vi "Periodic Tasks.vi"(8 "error in":errorcluster) -> ()   [LabVIEW 2013]
doc: "This VI runs in parallel to other tasks. It can contain as many user-defined periodic loops as you need. These can carry out PID or other sorts of timed response."
uses:
  <vilib>/Rock Robotics/WPI/Relay/WPI_RelayValue.ctl
  <vilib>/vision/Image Controls.llb/IMAQ Image.ctl
  <vilib>/Rock Robotics/SystemInterfaces/Utilities/FPGA_UtilitiesLED Source.ctl
  <vilib>/Rock Robotics/SystemInterfaces/Utilities/FPGA_UtilitiesLED State.ctl
  <vilib>/Rock Robotics/WPI/Solenoid/WPI_SolenoidValue.ctl
  Robot Global Data.vi
  <vilib>/Rock Robotics/WPI/Solenoid/WPI_SolenoidSetEnum.vi
  <vilib>/Rock Robotics/WPI/Joystick/WPI_JoystickGetSetRefNum.vi
  <vilib>/Rock Robotics/WPI/Solenoid/WPI_SolenoidGetEnum.vi
  <vilib>/Rock Robotics/WPI/Compressor/WPI_CompressorGetSetRefNum.vi
panel:
  out "Distance":dbl
  out "Rate 2":dbl
  out "Rate":dbl
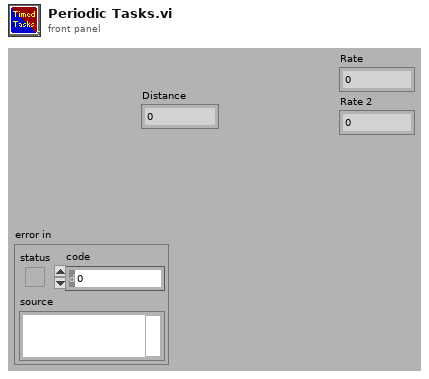
[diagram p1: front panel]
types:
  T1 = typedef "FPGA_UtilitiesLED State.ctl" = enum16{"Off", "On", "Toggle"}
  T2 = typedef "FPGA_UtilitiesLED Source.ctl" = enum16{"User LED", "FPGA LED"}
  T3 = typedef "WPI_DigitalInputDevRef.ctl" = cluster{"DevStatus":errorcluster, "DIO Channel":T4, "Digital Module":T5}
  T4 = typedef "FPGA_DIOChannel.ctl" = enum8{"DIO 1", "DIO 2", "DIO 3", "DIO 4", "DIO 5", "DIO 6", "DIO 7", "DIO 8", "DIO 9", "DIO 10", "DIO 11", "DIO 12", "DIO 13", "DIO 14", "Invalid"}
  T5 = typedef "FPGA_TypedefDigitalModule.ctl" = enum16{"Digital Module 1", "Digital Module 2"}
  T6 = typedef "WPI_SolenoidDevRef.ctl" = cluster{"DevStatus":errorcluster, "Solenoid Module":T7, "Forward Solenoid Channel":T8, "Reverse Solenoid Channel":T8}
  T7 = typedef "FPGA_TypedefSolenoidModule.ctl" = enum16{"Solenoid Module 1", "Solenoid Module 2"}
  T8 = typedef "WPI_SolenoidChannel.ctl" = enum8{"Solenoid 1", "Solenoid 2", "Solenoid 3", "Solenoid 4", "Solenoid 5", "Solenoid 6", "Solenoid 7", "Solenoid 8", "Invalid"}
  T9 = typedef "WPI_EncoderDevRef.ctl" = cluster{"DevStatus":errorcluster, "EncoderIndex":T10, "CounterIndex":T11, "DistancePerCount":dbl, "Decoding Type":T12}
  T10 = typedef "FPGA_EncoderIdx.ctl" = enum8{"Enc 0", "Enc 1", "Enc 2", "Enc 3", "Invalid"}
  T11 = typedef "FPGA_CounterCtrSystemIndex.ctl" = enum8{"Ctr 0", "Ctr 1", "Ctr 2", "Ctr 3", "Ctr 4", "Ctr 5", "Ctr 6", "Ctr 7", "Invalid"}
  T12 = typedef "WPI_EncoderType.ctl" = enum16{"1x", "2x", "4x"}
  T13 = typedef "WPI_JoystickDevRef.ctl" = cluster{"Device":T14}
  T14 = typedef "WPI_JoystickDeviceEnum.ctl" = enum16{"USB 1", "USB 2", "USB 3", "USB 4", "Kinect 1", "Kinect 2"}
  T15 = typedef "WPI_CompressorDevRef.ctl" = cluster{"DevStatus":errorcluster, "DigitalInputDevRef":T3, "RelayDevRef":T16}
  T16 = typedef "WPI_RelayDevRef.ctl" = cluster{"DevStatus":errorcluster, "Relay Channel":T17, "Digital Module":T5, "Relay Direction":T18}
  T17 = typedef "FPGA_DIORelayChannel.ctl" = enum8{"Relay 1", "Relay 2", "Relay 3", "Relay 4", "Relay 5", "Relay 6", "Relay 7", "Relay 8", "Invalid"}
  T18 = typedef "WPI_RelayDirection.ctl" = enum16{"Both directions", "Forward only", "Reverse only"}
  T19 = typedef "WPI_MotorControlDeviceRef.ctl" = cluster{"DeviceStatus":errorcluster, "Type":enum16{"PWM", "CAN"}, "PWM":cluster{"Digital Module":T5, "PWM Channel":T20, "DeadBand":T21}, "CAN":cluster{"Device Number":u8, "Control Mode":T22, "Semaphore":T23, "Max Vout":dbl}, "Invert":bool, "TransformRef":T24, "InvTransformRef":T24}
  T20 = typedef "FPGA_DIOPWMChannel.ctl" = enum8{"PWM 1", "PWM 2", "PWM 3", "PWM 4", "PWM 5", "PWM 6", "PWM 7", "PWM 8", "PWM 9", "PWM 10", "Invalid"}
  T21 = typedef "WPI_PWMDeadband.ctl" = cluster{"Name":string, "maxPositivePwm":i32, "minPositivePwm":i32, "centerPwm":i32, "maxNegativePwm":i32, "minNegativePwm":i32, "angularRange":u16}
  T22 = typedef "WPI_CANJaguar_ControlMode.ctl" = enum8{"Percent VBus", "Current", "Speed", "Position", "Voltage"}
  T23 = typedef "Semaphore RefNum" = refnum<k1>
  T24 = typedef "WPI_PWMTransform_ConPane.ctl" = refnum<vi>
  T25 = typedef "WPI_SolenoidValue.ctl" = enum16{"Off", "On", "Forward", "Reverse"}
  T26 = typedef "WPI_JoystickButtonState.ctl" = cluster{"Button 1":bool, "Button 2":bool, "Button 3":bool, "Button 4":bool, "Button 5":bool, "Button 6":bool, "Button 7":bool, "Button 8":bool, "Button 9":bool, "Button 10":bool, "Button 11":bool, "Button 12":bool}
  T27 = typedef "WPI_RelayValue.ctl" = enum16{"Off", "On", "Forward", "Reverse"}
  T28 = typedef "WPI_DriverStationPositionInfo.ctl" = enum16{"1", "2", "3"}
  T29 = typedef "WPI_DriverStationRobotMode2.ctl" = enum16{"Autonomous Disabled", "Autonomous Enabled", "Teleop Disabled", "Teleop Enabled", "Timeout", "Finish", "Test Disabled", "Test Enabled"}
  T30 = cluster{"Axes":cluster{"axis 1 (x)":dbl, "axis 2 (y)":dbl, "axis 3 (throttle)":dbl, "axis 4":dbl, "axis 5":dbl, "axis 6":dbl}, "Buttons":cluster{"Button 1":bool, "Button 2":bool, "Button 3":bool, "Button 4":bool, "Button 5":bool, "Button 6":bool, "Button 7":bool, "Button 8":bool, "Button 9":bool, "Button 10":bool, "Button 11":bool, "Button 12":bool}, "EncoderL":dbl, "EncoderR":dbl, "Down":bool, "Up":bool, "Up2":bool, "Down2":bool, "Center":bool, "Count":i32, "Region":i32}
  T31 = typedef "IMAQ Image.ctl" = refnum<image>
  T32 = cluster{"Axes":cluster{"axis 1 (x)":dbl, "axis 2 (y)":dbl, "axis 3 (throttle)":dbl, "axis 4":dbl, "axis 5":dbl, "axis 6":dbl}, "Buttons":cluster{"Button 1":bool, "Button 2":bool, "Button 3":bool, "Button 4":bool, "Button 5":bool, "Button 6":bool, "Button 7":bool, "Button 8":bool, "Button 9":bool, "Button 10":bool, "Button 11":bool, "Button 12":bool}, "Image":T31, "EncoderL":dbl, "EncoderR":dbl, "Down":bool, "Up":bool, "Up2":bool, "Down2":bool, "Center":bool, "Count":i32, "Region":i32}
  T33 = cluster{"Button 1":bool, "Button 2":bool, "Button 3":bool, "Button 4":bool, "Button 5":bool, "Button 6":bool, "Button 7":bool, "Button 8":bool, "Button 9":bool, "Button 10":bool, "Button 11":bool, "Button 12":bool}
  T34 = cluster{"axis 1 (x)":dbl, "axis 2 (y)":dbl, "axis 3 (throttle)":dbl, "axis 4":dbl, "axis 5":dbl, "axis 6":dbl}
  T35 = enum16{"ToPos2", "ToPos1", "Fire", "Wait", "ESTOP", "Reset", "ToLowPower", "ToHighPower"}
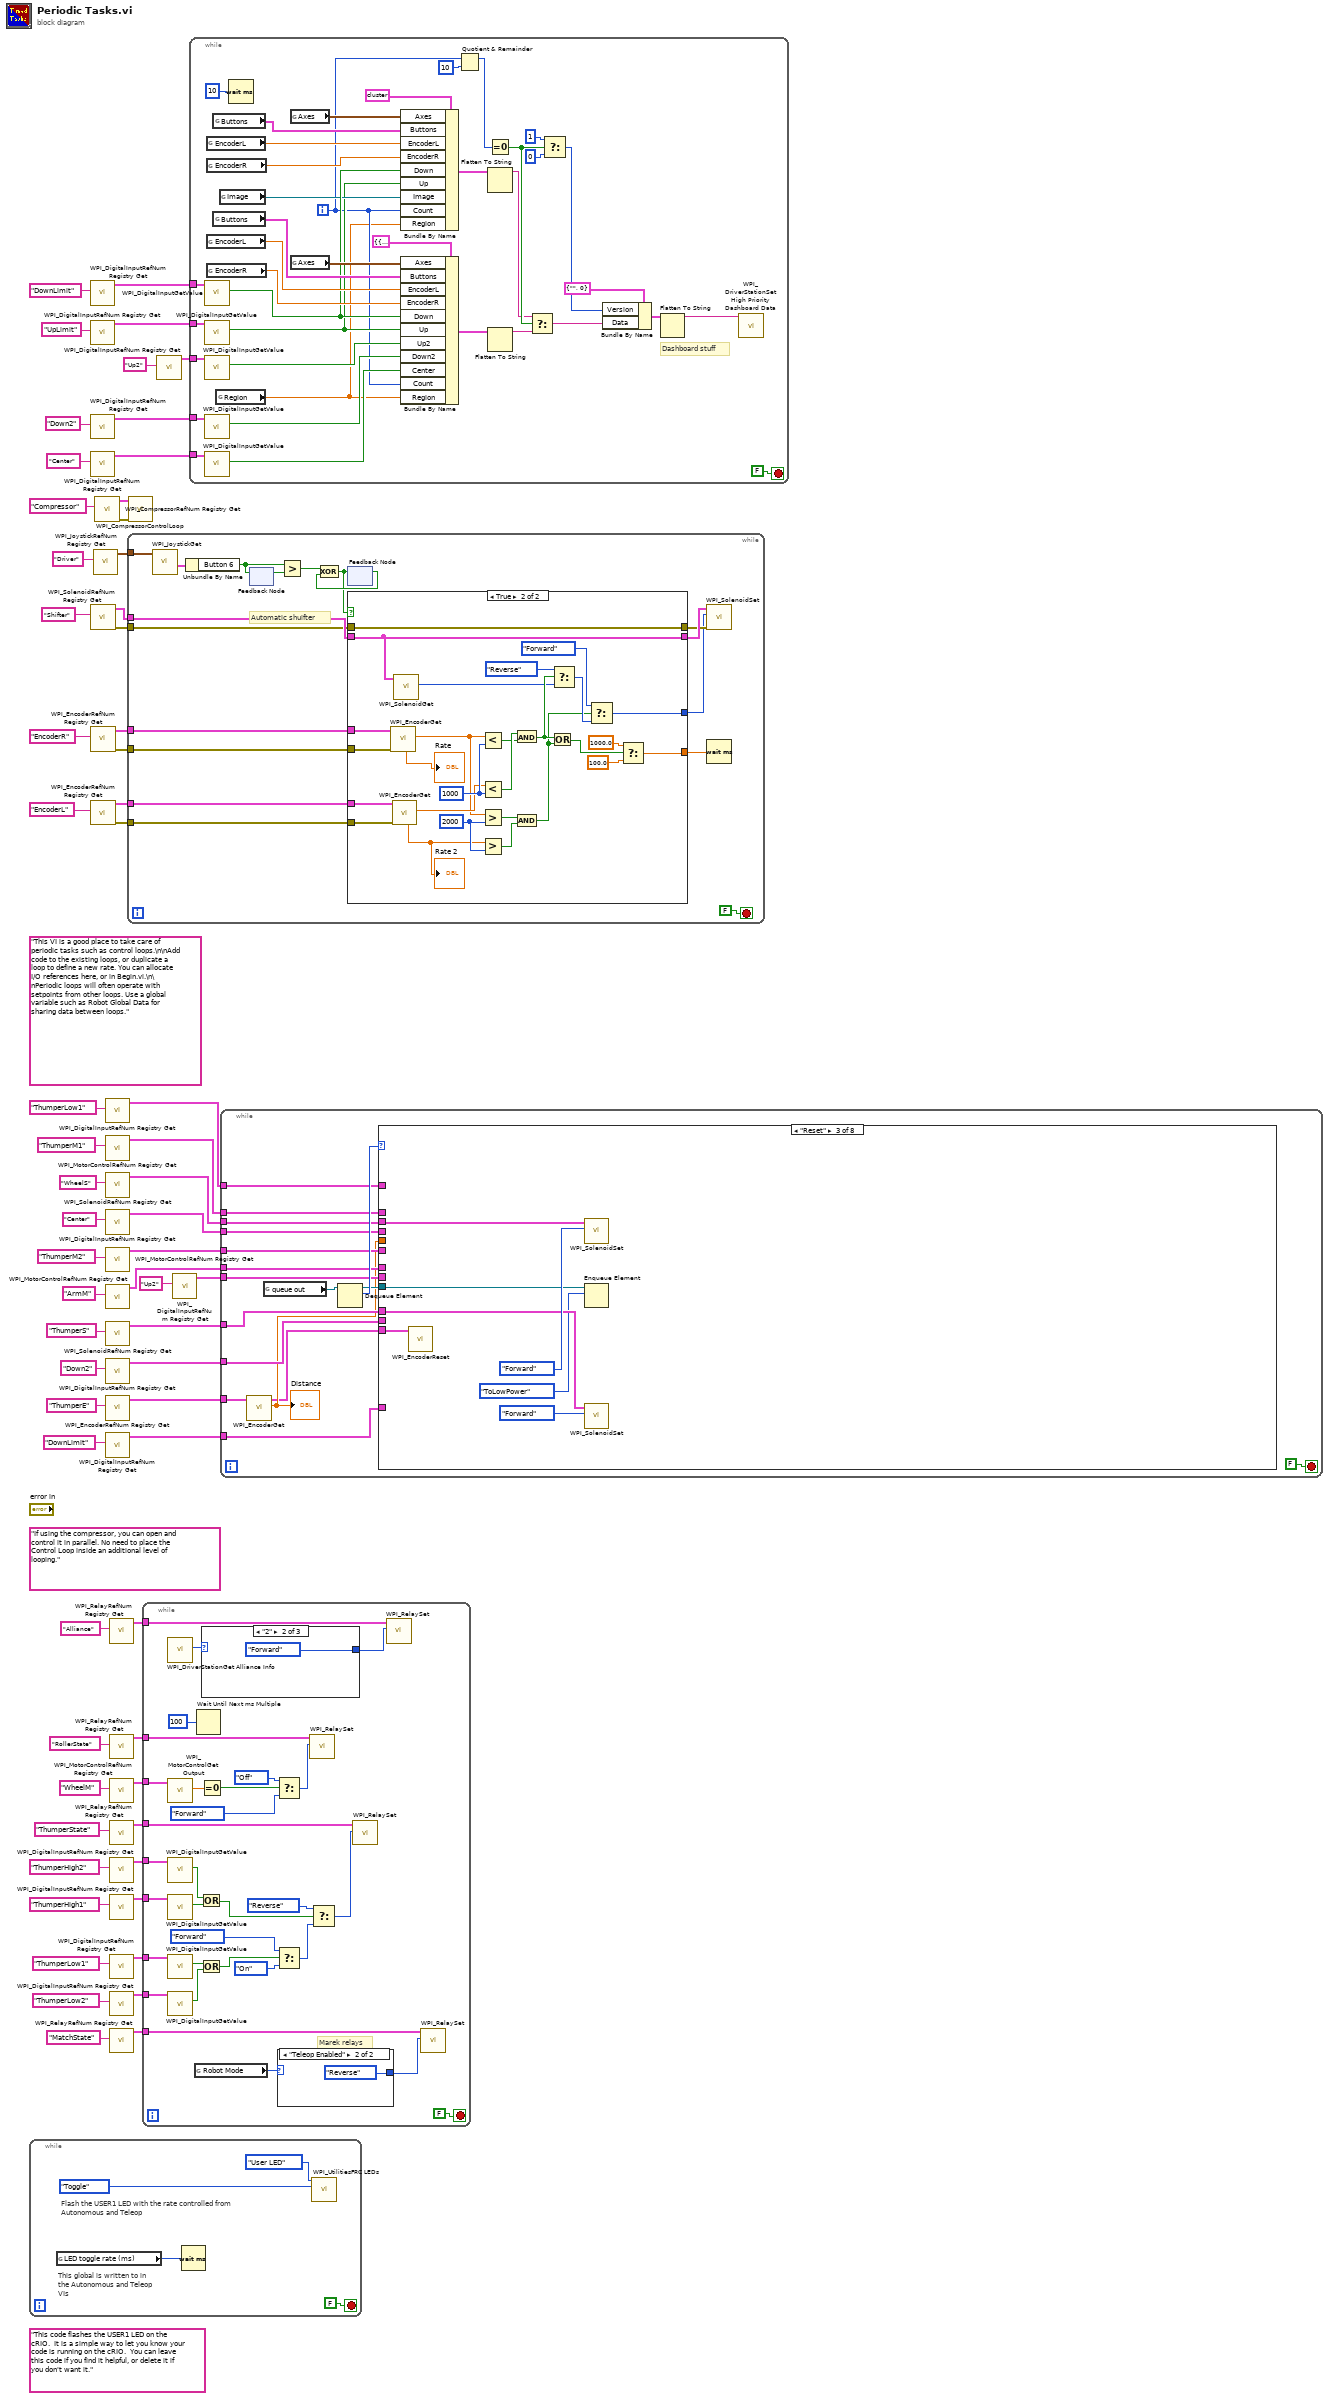
[diagram p0: block diagram]
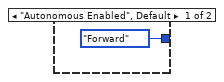
[diagram p2: hidden frame]
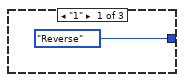
[diagram p3: hidden frame]
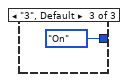
[diagram p4: hidden frame]
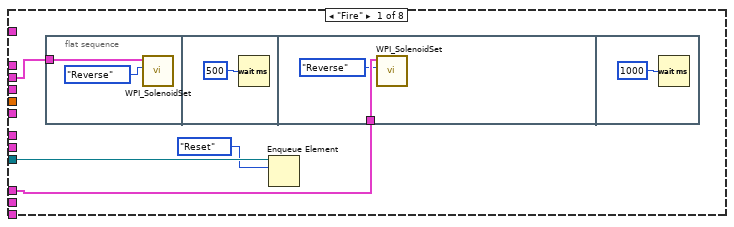
[diagram p5: hidden frame]
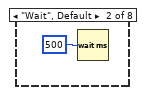
[diagram p6: hidden frame]
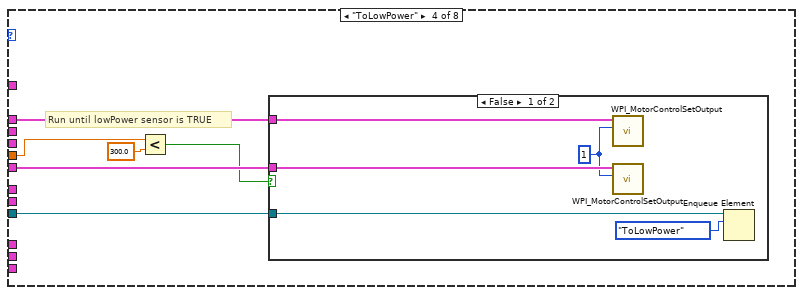
[diagram p7: hidden frame]
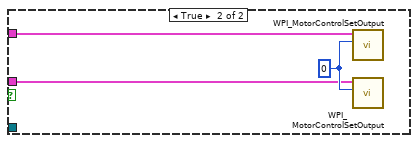
[diagram p8: hidden frame]
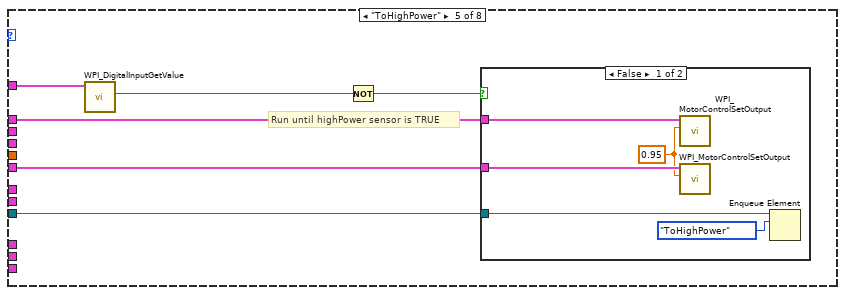
[diagram p9: hidden frame]
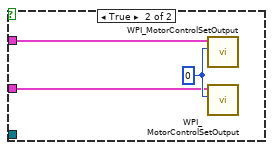
[diagram p10: hidden frame]
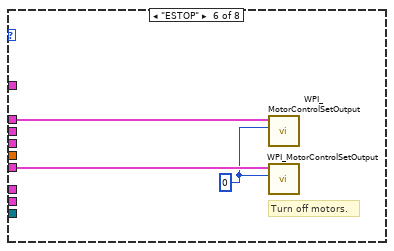
[diagram p11: hidden frame]
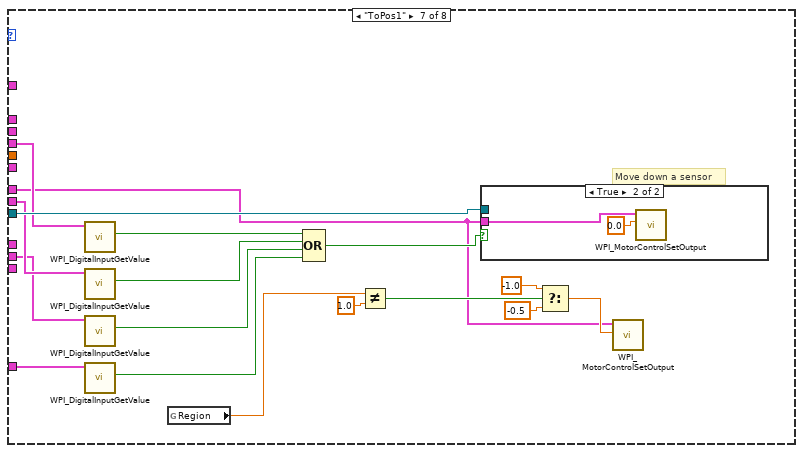
[diagram p12: hidden frame]
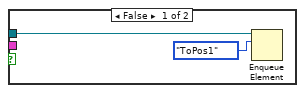
[diagram p13: hidden frame]
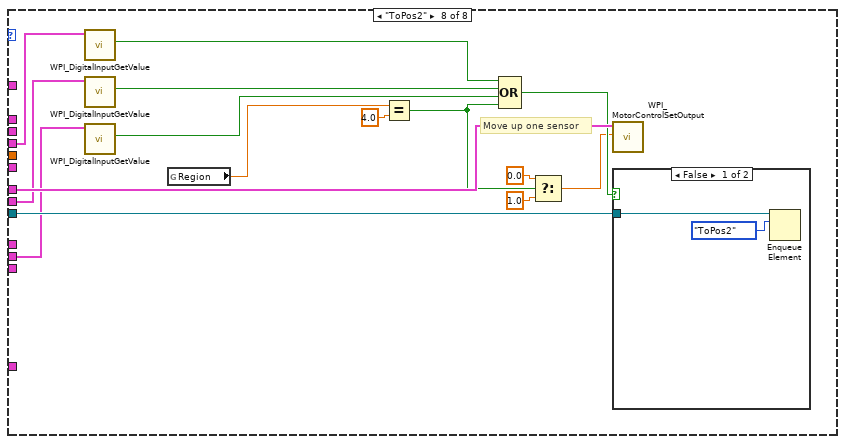
[diagram p14: hidden frame]
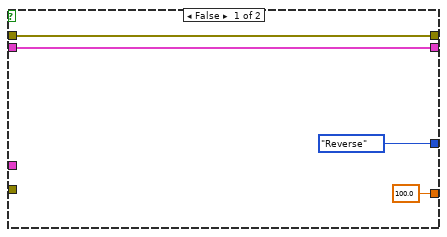
[diagram p16: hidden frame]
diagram:
  (unwired) "If using the compressor, you can open and control it in parallel. No need to place the Control Loop inside an additional level of looping."
  (unwired) "This code flashes the USER1 LED on the cRIO.  It is a simple way to let you know your code is running on the cRIO.  You can leave this code if you find it helpful, or delete it if you don't want it."
  (unwired) "This VI is a good place to take care of periodic tasks such as control loops.\n\nAdd code to the existing loops, or duplicate a loop to define a new rate. You can allocate I/O references here, or in Begin.vi.\n\nPeriodic loops will often operate with setpoints from other loops. Use a global variable such as Robot Global Data for sharing data between loops."
  n1 = while {
    stop <- FALSE stop-if-true
    # "This global is written to in the Autonomous and Teleop VIs"
    # "Flash the USER1 LED with the rate controlled from Autonomous and Teleop"
    n2 = global read "Robot Global Data.vi" "LED toggle rate (ms)"() -> (w65:u32)
    n3 = Wait (ms)(milliseconds to wait=w65) -> ()  [unwired: 1 out]
    n4 = call <vilib>:"WPI_UtilitiesFRC LEDs.vi"("State"=FPGA_UtilitiesLED_State."Toggle", "LED Type"=FPGA_UtilitiesLED_Source."User LED") -> ()  [unwired: 1 in, 9 out]
  }
  n5 = call <vilib>:"WPI_DigitalInputRefNum Registry Get.vi"("refnum name"="DownLimit") -> ("DigitalInputDevRef"=w48:T3)  [unwired: 9 in, 1 out]
  n6 = call <vilib>:"WPI_DigitalInputRefNum Registry Get.vi"("refnum name"="UpLimit") -> ("DigitalInputDevRef"=w47:T3)  [unwired: 9 in, 1 out]
  n7 = call <vilib>:"WPI_DigitalInputRefNum Registry Get.vi"("refnum name"="Down2") -> ("DigitalInputDevRef"=w6:T3)  [unwired: 9 in, 1 out]
  n8 = call <vilib>:"WPI_DigitalInputRefNum Registry Get.vi"("refnum name"="Center") -> ("DigitalInputDevRef"=w7:T3)  [unwired: 9 in, 1 out]
  n9 = call <vilib>:"WPI_SolenoidRefNum Registry Get.vi"("refnum name"="Shifter") -> ("error out"=w55:errorcluster, "SolenoidDevRef"=w56:T6)  [unwired: 9 in]
  n10 = call <vilib>:"WPI_EncoderRefNum Registry Get.vi"("refnum name"="EncoderR") -> ("error out"=w51:errorcluster, "EncoderDevRef"=w52:T9)  [unwired: 9 in]
  n11 = call <vilib>:"WPI_EncoderRefNum Registry Get.vi"("refnum name"="EncoderL") -> ("error out"=w53:errorcluster, "EncoderDevRef"=w54:T9)  [unwired: 9 in]
  n12 = call <vilib>:"WPI_JoystickRefNum Registry Get.vi"("refnum name"="Driver") -> ("JoystickDevRef"=w60:T13)  [unwired: 9 in, 1 out]
  n13 = call <vilib>:"WPI_CompressorRefNum Registry Get.vi"("refnum name"="Compressor") -> ("error out"=w62:errorcluster, "CompressorDevRef"=w63:T15)  [unwired: 9 in]
  n14 = call <vilib>:"WPI_DigitalInputRefNum Registry Get.vi"("refnum name"="ThumperLow1") -> ("DigitalInputDevRef"=w36:T3)  [unwired: 9 in, 1 out]
  n15 = call <vilib>:"WPI_MotorControlRefNum Registry Get.vi"("refnum name"="ThumperM1") -> ("MotorControlDevRef"=w37:T19)  [unwired: 9 in, 1 out]
  n16 = call <vilib>:"WPI_SolenoidRefNum Registry Get.vi"("refnum name"="WheelS") -> ("SolenoidDevRef"=w41:T6)  [unwired: 9 in, 1 out]
  n17 = call <vilib>:"WPI_DigitalInputRefNum Registry Get.vi"("refnum name"="Center") -> ("DigitalInputDevRef"=w3:T3)  [unwired: 9 in, 1 out]
  n18 = call <vilib>:"WPI_MotorControlRefNum Registry Get.vi"("refnum name"="ThumperM2") -> ("MotorControlDevRef"=w38:T19)  [unwired: 9 in, 1 out]
  n19 = call <vilib>:"WPI_MotorControlRefNum Registry Get.vi"("refnum name"="ArmM") -> ("MotorControlDevRef"=w39:T19)  [unwired: 9 in, 1 out]
  n20 = call <vilib>:"WPI_SolenoidRefNum Registry Get.vi"("refnum name"="ThumperS") -> ("SolenoidDevRef"=w40:T6)  [unwired: 9 in, 1 out]
  n21 = call <vilib>:"WPI_DigitalInputRefNum Registry Get.vi"("refnum name"="Down2") -> ("DigitalInputDevRef"=w34:T3)  [unwired: 9 in, 1 out]
  n22 = call <vilib>:"WPI_EncoderRefNum Registry Get.vi"("refnum name"="ThumperE") -> ("EncoderDevRef"=w30:T9)  [unwired: 9 in, 1 out]
  n23 = call <vilib>:"WPI_DigitalInputRefNum Registry Get.vi"("refnum name"="DownLimit") -> ("DigitalInputDevRef"=w1:T3)  [unwired: 9 in, 1 out]
  n24 = call <vilib>:"WPI_RelayRefNum Registry Get.vi"("refnum name"="Alliance") -> ("RelayDevRef"=w24:T16)  [unwired: 9 in, 1 out]
  n25 = call <vilib>:"WPI_RelayRefNum Registry Get.vi"("refnum name"="RollerState") -> ("RelayDevRef"=w23:T16)  [unwired: 9 in, 1 out]
  n26 = call <vilib>:"WPI_MotorControlRefNum Registry Get.vi"("refnum name"="WheelM") -> ("MotorControlDevRef"=w21:T19)  [unwired: 9 in, 1 out]
  n27 = call <vilib>:"WPI_RelayRefNum Registry Get.vi"("refnum name"="ThumperState") -> ("RelayDevRef"=w20:T16)  [unwired: 9 in, 1 out]
  n28 = call <vilib>:"WPI_DigitalInputRefNum Registry Get.vi"("refnum name"="ThumperHigh2") -> ("DigitalInputDevRef"=w15:T3)  [unwired: 9 in, 1 out]
  n29 = call <vilib>:"WPI_DigitalInputRefNum Registry Get.vi"("refnum name"="ThumperHigh1") -> ("DigitalInputDevRef"=w13:T3)  [unwired: 9 in, 1 out]
  n30 = call <vilib>:"WPI_DigitalInputRefNum Registry Get.vi"("refnum name"="ThumperLow1") -> ("DigitalInputDevRef"=w14:T3)  [unwired: 9 in, 1 out]
  n31 = call <vilib>:"WPI_DigitalInputRefNum Registry Get.vi"("refnum name"="ThumperLow2") -> ("DigitalInputDevRef"=w12:T3)  [unwired: 9 in, 1 out]
  n32 = call <vilib>:"WPI_RelayRefNum Registry Get.vi"("refnum name"="MatchState") -> ("RelayDevRef"=w11:T16)  [unwired: 9 in, 1 out]
  n33 = while {
    tunnel: w60 -> [w86]
    tunnel: w56 -> [w76]
    tunnel: w55 -> [w75]
    tunnel: w54 -> [w74]
    tunnel: w53 -> [w73]
    tunnel: w52 -> [w72]
    tunnel: w51 -> [w71]
    stop <- FALSE stop-if-true
    # "Automatic shuifter"
    n34 = call <vilib>:"WPI_JoystickGet.vi"("JoystickDevRef"=w86) -> ("Buttons"=w85:T26)  [unwired: 4 in, 2 out]
    n35 = Unbundle By Name(w85) -> ("Button 6"=w69:bool)
    n36 = feedback-in #1(w69) -> ()
    n37 = feedback #1() -> (w84:bool)  [unwired: 1 in]
    n38 = Greater?(x=w69, y=w84) -> (0:w83:bool)
    n39 = feedback #2() -> (w82:bool)  [unwired: 1 in]
    n40 = Exclusive Or(1:w82, 2:w83) -> (0:w81:bool)
    n41 = feedback-in #2(w81) -> ()
    n42 = case shown="True" w81 {
      tunnel: w74 -> [_ w117]
      tunnel: w73 -> [_ w116]
      tunnel: w72 -> [_ w115]
      tunnel: w71 -> [_ w114]
      tunnel: w76 -> [w89 w97]
      tunnel: w75 -> [w88 w106]
      tunnel: [w89 w97] -> w80
      tunnel: [w88 w106] -> w79
      tunnel: [WPI_SolenoidValue."Reverse" ("Value") w105] -> w78
      tunnel: [100.0 ("f") w101] -> w70
      frame False {
      }
      frame True {
        w113 = 2000
        w93 = 1000
        n43 = call <vilib>:"WPI_EncoderGet.vi"("error in (no error)"=w114, "EncoderDevRef"=w115) -> ("Distance"=w91:dbl, "Rate"=→"Rate":dbl)  [unwired: 4 in, 4 out]
        n44 = call <vilib>:"WPI_EncoderGet.vi"("error in (no error)"=w116, "EncoderDevRef"=w117) -> ("Distance"=w92:dbl, "Rate"=w94:dbl)  [unwired: 4 in, 4 out]
        "Rate 2" <- w94
        n45 = call-poly <vilib>:"WPI_SolenoidGet.vi"("SolenoidDevRef"=w97) -> ("Value"=w96:T25)  [unwired: 8 in, 2 out]
        n46 = Less?(x=w91, y=w93) -> (x < y?=w109:bool)
        n47 = Less?(x=w92, y=w93) -> (x < y?=w110:bool)
        n48 = Greater?(x=w91, y=w113) -> (0:w112:bool)
        n49 = Greater?(x=w94, y=w113) -> (0:w111:bool)
        n50 = And(x=w110, y=w109) -> (x .and. y?=w104:bool)
        n51 = And(x=w112, y=w111) -> (x .and. y?=w103:bool)
        n52 = Or(x=w104, y=w103) -> (x .or. y?=w102:bool)
        n53 = Select(t=WPI_SolenoidValue."Reverse" ("Value"), s=w104, f=w96) -> (s? t:f=w108:T25)
        n54 = Select(t=WPI_SolenoidValue."Forward" ("Value"), s=w103, f=w108) -> (s? t:f=w105:T25)
        n55 = Select(t=1000.0, s=w102, f=100.0) -> (s? t:f=w101:dbl)
      }
    }
    n56 = call-poly <vilib>:"WPI_SolenoidSet.vi"("error in (no error)"=w79, "Value"=w78, "SolenoidDevRef"=w80) -> ()  [unwired: 7 in, 2 out]
    n57 = Wait (ms)(milliseconds to wait=w70) -> ()  [unwired: 1 out]
  }
  n58 = call <vilib>:"WPI_CompressorControlLoop.vi"("error in (no error)"=w62, "CompressorDevRef"=w63) -> ()  [unwired: 10 in]
  n59 = while {
    tunnel: w24 -> [w146]
    tunnel: w23 -> [w144]
    tunnel: w21 -> [w143]
    tunnel: w20 -> [w137]
    tunnel: w15 -> [w136]
    tunnel: w14 -> [w135]
    tunnel: w13 -> [w134]
    tunnel: w12 -> [w133]
    tunnel: w11 -> [w121]
    stop <- FALSE stop-if-true
    # "Marek relays"
    n60 = call <vilib>:"WPI_DriverStationGet Alliance Info.vi"() -> ("Position"=w147:T28)  [unwired: 10 in, 1 out]
    n61 = call <vilib>:"WPI_MotorControlGetOutput.vi"("MotorControlDevRef"=w143) -> ("Output"=w142:dbl)  [unwired: 8 in, 2 out]
    n62 = call <vilib>:"WPI_DigitalInputGetValue.vi"("DigitalInputDevRef"=w136) -> ("Value"=w131:bool)  [unwired: 8 in, 2 out]
    n63 = call <vilib>:"WPI_DigitalInputGetValue.vi"("DigitalInputDevRef"=w134) -> ("Value"=w132:bool)  [unwired: 8 in, 2 out]
    n64 = call <vilib>:"WPI_DigitalInputGetValue.vi"("DigitalInputDevRef"=w135) -> ("Value"=w130:bool)  [unwired: 8 in, 2 out]
    n65 = call <vilib>:"WPI_DigitalInputGetValue.vi"("DigitalInputDevRef"=w133) -> ("Value"=w129:bool)  [unwired: 8 in, 2 out]
    n66 = global read "Robot Global Data.vi" "Robot Mode"() -> (w120:T29)
    n67 = Wait Until Next ms Multiple(millisecond multiple=u32 100) -> ()  [unwired: 1 out]
    n68 = Or(x=w131, y=w132) -> (x .or. y?=w128:bool)
    n69 = Or(x=w130, y=w129) -> (x .or. y?=w127:bool)
    n70 = Equal To 0?(x=w142) -> (x = 0?=w141:bool)
    n71 = case shown="\"2\"" w147 {
      tunnel: [WPI_RelayValue."Reverse" ("RelayValue") WPI_RelayValue."Forward" ("RelayValue") WPI_RelayValue."On" ("RelayValue")] -> w145
      frame "1" {
      }
      frame "2" {
      }
      frame "3", Default {
      }
    }
    n72 = Select(t=WPI_RelayValue."Off" ("RelayValue"), s=w141, f=WPI_RelayValue."Forward" ("RelayValue")) -> (s? t:f=w140:T27)
    n73 = Select(t=WPI_RelayValue."Forward" ("RelayValue"), s=w127, f=WPI_RelayValue."On" ("RelayValue")) -> (s? t:f=w125:T27)
    n74 = case shown="\"Teleop Enabled\"" w120 {
      tunnel: [WPI_RelayValue."Forward" ("RelayValue") WPI_RelayValue."Reverse" ("RelayValue")] -> w119
      frame "Autonomous Enabled", Default {
      }
      frame "Teleop Enabled" {
      }
    }
    n75 = call <vilib>:"WPI_RelaySet.vi"("RelayValue"=w140, "RelayDevRef"=w144) -> ()  [unwired: 8 in, 2 out]
    n76 = Select(t=WPI_RelayValue."Reverse" ("RelayValue"), s=w128, f=w125) -> (s? t:f=w124:T27)
    n77 = call <vilib>:"WPI_RelaySet.vi"("RelayValue"=w124, "RelayDevRef"=w137) -> ()  [unwired: 8 in, 2 out]
    n78 = call <vilib>:"WPI_RelaySet.vi"("RelayValue"=w145, "RelayDevRef"=w146) -> ()  [unwired: 8 in, 2 out]
    n79 = call <vilib>:"WPI_RelaySet.vi"("RelayValue"=w119, "RelayDevRef"=w121) -> ()  [unwired: 8 in, 2 out]
  }
  n80 = call <vilib>:"WPI_DigitalInputRefNum Registry Get.vi"("refnum name"="Up2") -> ("DigitalInputDevRef"=w5:T3)  [unwired: 9 in, 1 out]
  n81 = call <vilib>:"WPI_DigitalInputRefNum Registry Get.vi"("refnum name"="Up2") -> ("DigitalInputDevRef"=w32:T3)  [unwired: 9 in, 1 out]
  n82 = while {
    tunnel: w48 -> [w164]
    tunnel: w47 -> [w163]
    tunnel: w7 -> [w162]
    tunnel: w6 -> [w161]
    tunnel: w5 -> [w160]
    i -> [w156]
    stop <- FALSE stop-if-true
    # "Dashboard stuff"
    n83 = call <vilib>:"WPI_DigitalInputGetValue.vi"("DigitalInputDevRef"=w164) -> ("Value"=w172:bool)  [unwired: 8 in, 2 out]
    n84 = call <vilib>:"WPI_DigitalInputGetValue.vi"("DigitalInputDevRef"=w163) -> ("Value"=w170:bool)  [unwired: 8 in, 2 out]
    n85 = call <vilib>:"WPI_DigitalInputGetValue.vi"("DigitalInputDevRef"=w160) -> ("Value"=w159:bool)  [unwired: 8 in, 2 out]
    n86 = call <vilib>:"WPI_DigitalInputGetValue.vi"("DigitalInputDevRef"=w161) -> ("Value"=w158:bool)  [unwired: 8 in, 2 out]
    n87 = call <vilib>:"WPI_DigitalInputGetValue.vi"("DigitalInputDevRef"=w162) -> ("Value"=w157:bool)  [unwired: 8 in, 2 out]
    n88 = global read "Robot Global Data.vi" "EncoderL"() -> (w181:dbl)
    n89 = global read "Robot Global Data.vi" "EncoderR"() -> (w180:dbl)
    n90 = global read "Robot Global Data.vi" "EncoderL"() -> (w187:dbl)
    n91 = global read "Robot Global Data.vi" "EncoderR"() -> (w186:dbl)
    n92 = global read "Robot Global Data.vi" "Buttons"() -> (w183:T33)
    n93 = global read "Robot Global Data.vi" "Buttons"() -> (w189:T33)
    n94 = global read "Robot Global Data.vi" "Region"() -> (w154:dbl)
    n95 = global read "Robot Global Data.vi" "Image"() -> (w171:T31)
    n96 = Wait (ms)(milliseconds to wait=u32 10) -> ()  [unwired: 1 out]
    n97 = global read "Robot Global Data.vi" "Axes"() -> (w184:T34)
    n98 = global read "Robot Global Data.vi" "Axes"() -> (w190:T34)
    n99 = Bundle By Name(cluster=T32 {"Axes"={"axis 1 (x)"=0.0, "axis 2 (y)"=0.0, "axis 3 (throttle)"=0.0, "axis 4"=0.0, "axis 5"=0.0, "axis 6"=0.0}, "Buttons"={"Button 1"=FALSE, "Button 2"=FALSE, "Button 3"=FALSE, "Button 4"=FALSE, "Button 5"=FALSE, "Button 6"=FALSE, "Button 7"=FALSE, "Button 8"=FALSE, "Button 9"=FALSE, "Button 10"=FALSE, "Button 11"=FALSE, "Button 12"=FALSE}, "Image"=refnum, "EncoderL"=0.0, "EncoderR"=0.0, "Down"=FALSE, "Up"=TRUE, "Up2"=TRUE, "Down2"=TRUE, "Center"=TRUE, "Count"=0, "Region"=0}, "Axes"=w184, "Buttons"=w183, "EncoderL"=w181, "EncoderR"=w180, "Down"=w172, "Up"=w170, "Image"=w171, "Count"=w156, "Region"=w154) -> (w182:T32)
    n100 = Bundle By Name(cluster=T30 {"Axes"={"axis 1 (x)"=0.0, "axis 2 (y)"=0.0, "axis 3 (throttle)"=0.0, "axis 4"=0.0, "axis 5"=0.0, "axis 6"=0.0}, "Buttons"={"Button 1"=FALSE, "Button 2"=FALSE, "Button 3"=FALSE, "Button 4"=FALSE, "Button 5"=FALSE, "Button 6"=FALSE, "Button 7"=FALSE, "Button 8"=FALSE, "Button 9"=FALSE, "Button 10"=FALSE, "Button 11"=FALSE, "Button 12"=FALSE}, "EncoderL"=0.0, "EncoderR"=0.0, "Down"=FALSE, "Up"=TRUE, "Up2"=TRUE, "Down2"=TRUE, "Center"=TRUE, "Count"=0, "Region"=0}, "Axes"=w190, "Buttons"=w189, "EncoderL"=w187, "EncoderR"=w186, "Down"=w172, "Up"=w170, "Up2"=w159, "Down2"=w158, "Center"=w157, "Count"=w156, "Region"=w154) -> (w188:T30)
    n101 = Quotient & Remainder(x=w156, y=10) -> (x-y*floor(x/y)=w178:i32)  [unwired: 1 out]
    n102 = Equal To 0?(x=w178) -> (x = 0?=w173:bool)
    n103 = Flatten To String(anything=w182) -> (data string=w165:string)  [unwired: 3 in, 2 out]
    n104 = Flatten To String(anything=w188) -> (data string=w166:string)  [unwired: 3 in, 2 out]
    n105 = Select(t=w165, s=w173, f=w166) -> (s? t:f=w169:string)
    n106 = Select(t=1, s=w173, f=0) -> (s? t:f=w174:i32)
    n107 = Bundle By Name(cluster=cluster{"Data":string, "Version":i32} {"Data"="", "Version"=0} ("input cluster"), "Version"=w174, "Data"=w169) -> (w168:cluster{"Data":string, "Version":i32})
    n108 = Flatten To String(anything=w168) -> (data string=w167:string)  [unwired: 3 in, 2 out]
    n109 = call <vilib>:"WPI_DriverStationSet High Priority Dashboard Data.vi"("User Data"=w167) -> ()  [unwired: 10 in, 1 out]
  }
  n110 = while {
    tunnel: w41 -> [w205]
    tunnel: w40 -> [w204]
    tunnel: w39 -> [w203]
    tunnel: w38 -> [w202]
    tunnel: w37 -> [w201]
    tunnel: w36 -> [w198]
    tunnel: w34 -> [w200]
    tunnel: w32 -> [w199]
    tunnel: w30 -> [w197]
    tunnel: w3 -> [w195]
    tunnel: w1 -> [w194]
    stop <- FALSE stop-if-true
    n111 = call <vilib>:"WPI_EncoderGet.vi"("EncoderDevRef"=w197) -> ("Distance"=w196:dbl, "EncoderDevRef"=w193:T9)  [unwired: 5 in, 4 out]
    "Distance" <- w196
    n112 = global read "Robot Global Data.vi" "queue out"() -> (w209:refnum<queue>)
    n113 = Dequeue Element(queue=w209) -> (queue out=w206:refnum<queue>, element=w207:T35)  [unwired: 2 in, 2 out]
    n114 = case shown="\"Reset\"" w207 {
      tunnel: w205 -> [w213 _ w226 _ _ _ _ _]
      tunnel: w204 -> [w212 _ w224 _ _ _ _ _]
      tunnel: w206 -> [w211 _ w223 w231 w245 _ w275 w293]
      tunnel: w202 -> [_ _ _ w233 w247 w257 _ _]
      tunnel: w201 -> [_ _ _ w232 w246 w258 _ _]
      tunnel: w203 -> [_ _ _ _ _ _ w259 w294]
      tunnel: w200 -> [_ _ _ _ _ _ w273 w292]
      tunnel: w199 -> [_ _ _ _ _ _ w274 w290]
      tunnel: w198 -> [_ _ _ _ w243 _ _ _]
      tunnel: w196 -> [_ _ _ w229 _ _ _ _]
      tunnel: w195 -> [_ _ _ _ _ _ w272 w291]
      tunnel: w194 -> [_ _ _ _ _ _ w271 _]
      tunnel: w193 -> [_ _ w221 _ _ _ _ _]
      frame "Fire" {
        n115 = flat-sequence {
          tunnel: w213 -> [w215]
          tunnel: w212 -> [w218]
          frame #0 {
            n116 = call-poly <vilib>:"WPI_SolenoidSet.vi"("Value"=WPI_SolenoidValue."Reverse", "SolenoidDevRef"=w215) -> ()  [unwired: 8 in, 2 out]
          }
          frame #1 {
            n117 = Wait (ms)(milliseconds to wait=u32 500) -> ()  [unwired: 1 out]
          }
          frame #2 {
            n118 = call-poly <vilib>:"WPI_SolenoidSet.vi"("Value"=WPI_SolenoidValue."Reverse", "SolenoidDevRef"=w218) -> ()  [unwired: 8 in, 2 out]
          }
          frame #3 {
            n119 = Wait (ms)(milliseconds to wait=u32 1000) -> ()  [unwired: 1 out]
          }
        }
        n120 = Enqueue Element(queue=w211, element=T35."Reset") -> ()  [unwired: 2 in, 3 out]
      }
      frame "Wait", Default {
        n121 = Wait (ms)(milliseconds to wait=u32 500) -> ()  [unwired: 1 out]
      }
      frame "Reset" {
        n122 = call <vilib>:"WPI_EncoderReset.vi"("EncoderDevRef"=w221) -> ()  [unwired: 9 in, 2 out]
        n123 = call-poly <vilib>:"WPI_SolenoidSet.vi"("Value"=WPI_SolenoidValue."Forward", "SolenoidDevRef"=w226) -> ()  [unwired: 8 in, 2 out]
        n124 = Enqueue Element(queue=w223, element=T35."ToLowPower") -> ()  [unwired: 2 in, 3 out]
        n125 = call-poly <vilib>:"WPI_SolenoidSet.vi"("Value"=WPI_SolenoidValue."Forward", "SolenoidDevRef"=w224) -> ()  [unwired: 8 in, 2 out]
      }
      frame "ToLowPower" {
        # "Run until lowPower sensor is TRUE"
        n126 = Less?(x=w229, y=300.0) -> (x < y?=w230:bool)
        n127 = case shown="False" w230 {
          tunnel: w233 -> [w238 w240]
          tunnel: w232 -> [w237 w239]
          tunnel: w231 -> [w235 _]
          frame False {
            w236 = 1
            n128 = call <vilib>:"WPI_MotorControlSetOutput.vi"("Output"=w236, "MotorControlDevRef"=w237) -> ()  [unwired: 7 in, 3 out]
            n129 = call <vilib>:"WPI_MotorControlSetOutput.vi"("Output"=w236, "MotorControlDevRef"=w238) -> ()  [unwired: 7 in, 3 out]
            n130 = Enqueue Element(queue=w235, element=T35."ToLowPower") -> ()  [unwired: 2 in, 3 out]
          }
          frame True {
            w241 = 0
            n131 = call <vilib>:"WPI_MotorControlSetOutput.vi"("Output"=w241, "MotorControlDevRef"=w239) -> ()  [unwired: 7 in, 3 out]
            n132 = call <vilib>:"WPI_MotorControlSetOutput.vi"("Output"=w241, "MotorControlDevRef"=w240) -> ()  [unwired: 7 in, 3 out]
          }
        }
      }
      frame "ToHighPower" {
        # "Run until highPower sensor is TRUE"
        n133 = call <vilib>:"WPI_DigitalInputGetValue.vi"("DigitalInputDevRef"=w243) -> ("Value"=w244:bool)  [unwired: 8 in, 2 out]
        n134 = Not(x=w244) -> (.not. x?=w242:bool)
        n135 = case shown="False" w242 {
          tunnel: w247 -> [w252 w254]
          tunnel: w246 -> [w251 w253]
          tunnel: w245 -> [w249 _]
          frame False {
            w250 = 0.95
            n136 = call <vilib>:"WPI_MotorControlSetOutput.vi"("Output"=w250, "MotorControlDevRef"=w251) -> ()  [unwired: 7 in, 3 out]
            n137 = call <vilib>:"WPI_MotorControlSetOutput.vi"("Output"=w250, "MotorControlDevRef"=w252) -> ()  [unwired: 7 in, 3 out]
            n138 = Enqueue Element(queue=w249, element=T35."ToHighPower") -> ()  [unwired: 2 in, 3 out]
          }
          frame True {
            w255 = 0
            n139 = call <vilib>:"WPI_MotorControlSetOutput.vi"("Output"=w255, "MotorControlDevRef"=w253) -> ()  [unwired: 7 in, 3 out]
            n140 = call <vilib>:"WPI_MotorControlSetOutput.vi"("Output"=w255, "MotorControlDevRef"=w254) -> ()  [unwired: 7 in, 3 out]
          }
        }
      }
      frame "ESTOP" {
        w256 = 0
        # "Turn off motors."
        n141 = call <vilib>:"WPI_MotorControlSetOutput.vi"("Output"=w256, "MotorControlDevRef"=w258) -> ()  [unwired: 7 in, 3 out]
        n142 = call <vilib>:"WPI_MotorControlSetOutput.vi"("Output"=w256, "MotorControlDevRef"=w257) -> ()  [unwired: 7 in, 3 out]
      }
      frame "ToPos1" {
        # "Move down a sensor"
        n143 = call <vilib>:"WPI_DigitalInputGetValue.vi"("DigitalInputDevRef"=w272) -> ("Value"=w269:bool)  [unwired: 8 in, 2 out]
        n144 = call <vilib>:"WPI_DigitalInputGetValue.vi"("DigitalInputDevRef"=w274) -> ("Value"=w268:bool)  [unwired: 8 in, 2 out]
        n145 = call <vilib>:"WPI_DigitalInputGetValue.vi"("DigitalInputDevRef"=w273) -> ("Value"=w267:bool)  [unwired: 8 in, 2 out]
        n146 = call <vilib>:"WPI_DigitalInputGetValue.vi"("DigitalInputDevRef"=w271) -> ("Value"=w266:bool)  [unwired: 8 in, 2 out]
        n147 = global read "Robot Global Data.vi" "Region"() -> (w265:dbl)
        n148 = Compound Arithmetic op=OR(w269, w268, w267, w266) -> (w270:bool)
        n149 = Not Equal?(x=w265, y=1.0) -> (x != y?=w263:bool)
        n150 = case shown="True" w270 {
          tunnel: w275 -> [w276 _]
          tunnel: w259 -> [_ w279]
          frame False {
            n151 = Enqueue Element(queue=w276, element=T35."ToPos1") -> ()  [unwired: 2 in, 3 out]
          }
          frame True {
            n152 = call <vilib>:"WPI_MotorControlSetOutput.vi"("Output"=0.0, "MotorControlDevRef"=w279) -> ()  [unwired: 7 in, 3 out]
          }
        }
        n153 = Select(t=-1.0, s=w263, f=-0.5) -> (s? t:f=w260:dbl)
        n154 = call <vilib>:"WPI_MotorControlSetOutput.vi"("Output"=w260, "MotorControlDevRef"=w259) -> ()  [unwired: 7 in, 3 out]
      }
      frame "ToPos2" {
        # "Move up one sensor"
        n155 = call <vilib>:"WPI_DigitalInputGetValue.vi"("DigitalInputDevRef"=w291) -> ("Value"=w289:bool)  [unwired: 8 in, 2 out]
        n156 = call <vilib>:"WPI_DigitalInputGetValue.vi"("DigitalInputDevRef"=w290) -> ("Value"=w288:bool)  [unwired: 8 in, 2 out]
        n157 = call <vilib>:"WPI_DigitalInputGetValue.vi"("DigitalInputDevRef"=w292) -> ("Value"=w287:bool)  [unwired: 8 in, 2 out]
        n158 = global read "Robot Global Data.vi" "Region"() -> (w285:dbl)
        n159 = Equal?(x=w285, y=4.0) -> (x = y?=w283:bool)
        n160 = Compound Arithmetic op=OR(w289, w288, w287, w283) -> (w286:bool)
        n161 = Select(t=0.0, s=w283, f=1.0) -> (s? t:f=w280:dbl)
        n162 = call <vilib>:"WPI_MotorControlSetOutput.vi"("Output"=w280, "MotorControlDevRef"=w294) -> ()  [unwired: 7 in, 3 out]
        n163 = case shown="False" w286 {
          tunnel: w293 -> [w295 _]
          frame False {
            n164 = Enqueue Element(queue=w295, element=T35."ToPos2") -> ()  [unwired: 2 in, 3 out]
          }
          frame True {
          }
        }
      }
    }
  }
